vi "convertColorIntoLetter.vi"(11 "Array":string[](array[string])) -> (2 "String":string)   [LabVIEW 2019]
uses:
  <vilib>/regexp/Match Regular Expression.xnode
panel:
  out "spreadsheet string":string
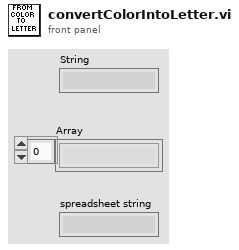
[diagram p1: front panel]
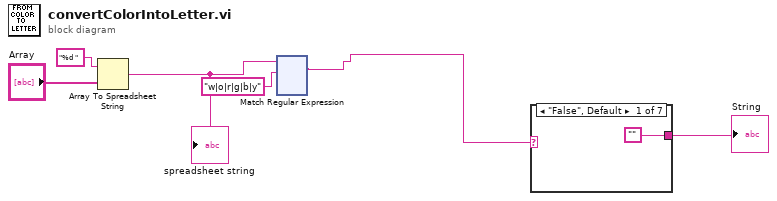
[diagram p0: block diagram]
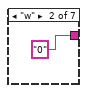
[diagram p2: hidden frame]
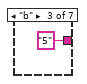
[diagram p3: hidden frame]
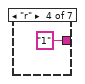
[diagram p4: hidden frame]
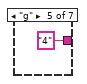
[diagram p5: hidden frame]
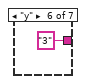
[diagram p6: hidden frame]
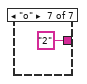
[diagram p7: hidden frame]
diagram:
  n1 = Array To Spreadsheet String(array="Array", 3:"%d " ("format string")) -> (spreadsheet string=w4:string)  [unwired: 1 in]
  "spreadsheet string" <- w4
  n2 = xnode "Match Regular Expression"("input string"=w4, "regular expression"="w|o|r|g|b|y" ("input string")) -> ("whole match"=w1:string)  [unwired: 4 in, 4 out]
  n3 = case shown="\"False\", Default" w1 {
    tunnel: ["" "0" "5" "1" "4" "3" "2"] -> w2
    frame "False", Default {
    }
    frame "w" {
    }
    frame "b" {
    }
    frame "r" {
    }
    frame "g" {
    }
    frame "y" {
    }
    frame "o" {
    }
  }
  "String" <- w2
